vi "Line Configuration Dialog.vi"(8 "error in":errorcluster, 9 "engine configuration in":refnum<class "engine configuration.lvclass">, 10 "tag bus configurable plugin module configuration":refnum<class "OPC UA Client configuration.lvclass">, 11 "Line":T4 {"OPC UA Data Type" items=["Boolean"=1, "SByte"=2, "Byte"=3, "Int16"=4, "UInt16"=5, "Int32"=6, "UInt32"=7, "Int64"=8, "UInt64"=9, "Float"=10, "Double"=11, "String"=12, "DateTime"=13, "ByteString"=15, "Array of Boolean"=101, "Array of SByte"=102, "Array of Byte"=103, "Array of Int16"=104, "Array of UInt16"=105, "Array of Int32"=106, "Array of UInt32"=107, "Array of Int64"=108, "Array of UInt64"=109, "Array of Float"=110, "Array of Double"=111, "Array of String"=112, "Array of DateTime"=113, "Array of ByteString"=115]}) -> (0 "error out":errorcluster, 1 "success":bool, 2 "changed":bool, 3 "Mappings out":T3 {"Line"."OPC UA Data Type" items=["Boolean"=1, "SByte"=2, "Byte"=3, "Int16"=4, "UInt16"=5, "Int32"=6, "UInt32"=7, "Int64"=8, "UInt64"=9, "Float"=10, "Double"=11, "String"=12, "DateTime"=13, "ByteString"=15, "Array of Boolean"=101, "Array of SByte"=102, "Array of Byte"=103, "Array of Int16"=104, "Array of UInt16"=105, "Array of Int32"=106, "Array of UInt32"=107, "Array of Int64"=108, "Array of UInt64"=109, "Array of Float"=110, "Array of Double"=111, "Array of String"=112, "Array of DateTime"=113, "Array of ByteString"=115]})   [LabVIEW 2014, in "OPC UA Client editor node.lvclass"]
uses:
  OPC UA Client editor node.lvclass
  module/configuration/Line.ctl
  <vilib>/NI/Tag Bus Module Framework/channel/TBM channel.lvclass
  module/configuration/OPC UA Data Type.ctl
  Mappings.ctl
  Map.ctl
  permissions.ctl
  <vilib>/NI/Module Execution Interface/Engine Configuration/engine configuration.lvclass
  module/configuration/OPC UA Client configuration.lvclass
  OPC UA DataType Enum.ctl
  <vilib>/NI/Tag Bus Module Framework/channel/TBM channel.lvclass/TBM channel.ctl
  <vilib>/NI/Configuration Framework/serializable configuration/NISE_CEF_serializable configuration.lvclass/NISE_CEF_serializable configuration.ctl
  <vilib>/NI/Tag Bus/tag/tag descriptor.lvclass/tag descriptor.ctl
  <vilib>/NI/Tag Bus/tag/write tag name.vi
  <vilib>/NI/Tag Bus Module Framework/channel/Write channel classification.vi
  <vilib>/NI/Tag Bus/tag/write data type.vi
  <vilib>/NI/Configuration Framework/serializable configuration/Read UID.vi
  <vilib>/NI/Tag Bus Module Framework/channel/Read channel classification.vi
  <vilib>/Utility/LVClass/Get LV Class Name.vi
  <vilib>/NI/Configuration Framework/error generator/NISE_error generator.vi
  <vilib>/NI/Tag Bus/tag/tag descriptor.lvclass
panel:
  in  "OPC Data Type":T1
  in  "Node Path":string="Channel_0"
  out "errors":string
  in  "Access Type":T2
  in  "Tag":i32(listbox)
  in  "Data Type":i32(listbox)
  in  "cancel":bool
  in  "ok":bool
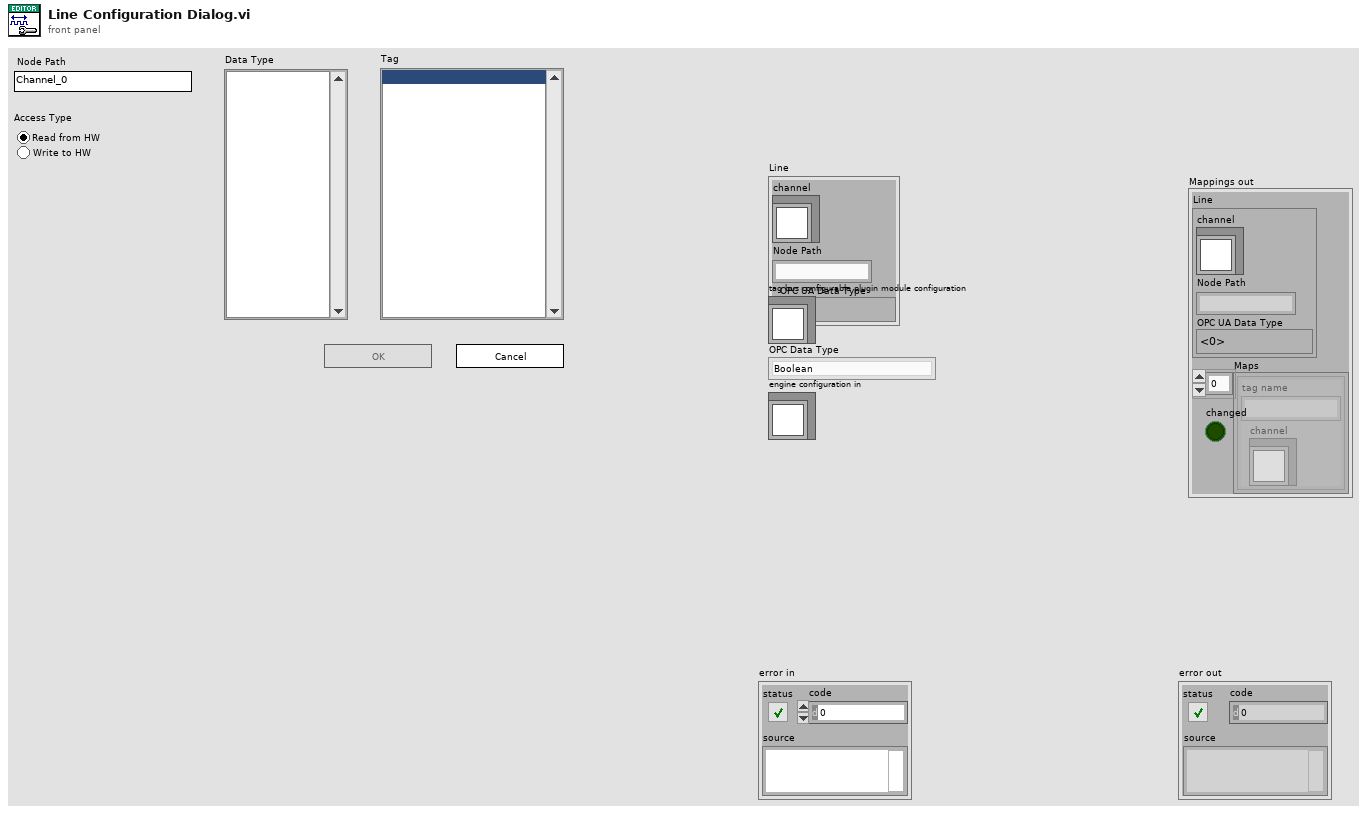
[diagram p1: front panel]
types:
  T1 = typedef "OPC UA Client editor node.lvclass/OPC UA DataType Enum.ctl" = enum16{"Boolean", "SByte", "Byte", "Int16", "UInt16", "Int32", "UInt32", "Int64", "UInt64", "Float", "Double", "String", "DateTime", "ByteString", "Array of Boolean", "Array of SByte", "Array of Byte", "Array of Int16", "Array of UInt16", "Array of Int32", "Array of UInt32", "Array of Int64", "Array of UInt64", "Array of Float", "Array of Double", "Array of String", "Array of DateTime"}
  T2 = typedef "OPC UA Client editor node.lvclass/permissions.ctl" = enum32{"Read from HW", "Write to HW"}
  T3 = typedef "OPC UA Client editor node.lvclass/Mappings.ctl" = cluster{"Line":T4, "Maps":T6[]}
  T4 = typedef "OPC UA Client configuration.lvclass/Line.ctl" = cluster{"channel":refnum<class "TBM channel.lvclass">, "Node Path":string, "OPC UA Data Type":T5}
  T5 = typedef "OPC UA Client configuration.lvclass/OPC UA Data Type.ctl" = u16
  T6 = typedef "OPC UA Client editor node.lvclass/Map.ctl" = cluster{"channel":refnum<class "TBM channel.lvclass">, "tag name":string}
  T7 = typedef "TBM channel.lvclass/channel classification.ctl" = enum16{"input data", "output data", "processing parameter", "processing result"}
  T8 = enum8{"Enabled", "Disabled", "Disabled and Grayed Out"}
  T9 = typedef "tag bus.lvlib/tag descriptor.lvclass/Data Type.ctl" = enum16{"Double", "Single", "I64", "I32", "I16", "I8", "U64", "U32", "U16", "U8", "Boolean", "String", "Array of Double", "Array of Single", "Array of I64", "Array of I32", "Array of I16", "Array of I8", "Array of U64", "Array of U32", "Array of U16", "Array of U8", "Array of Boolean", "Array of String"}
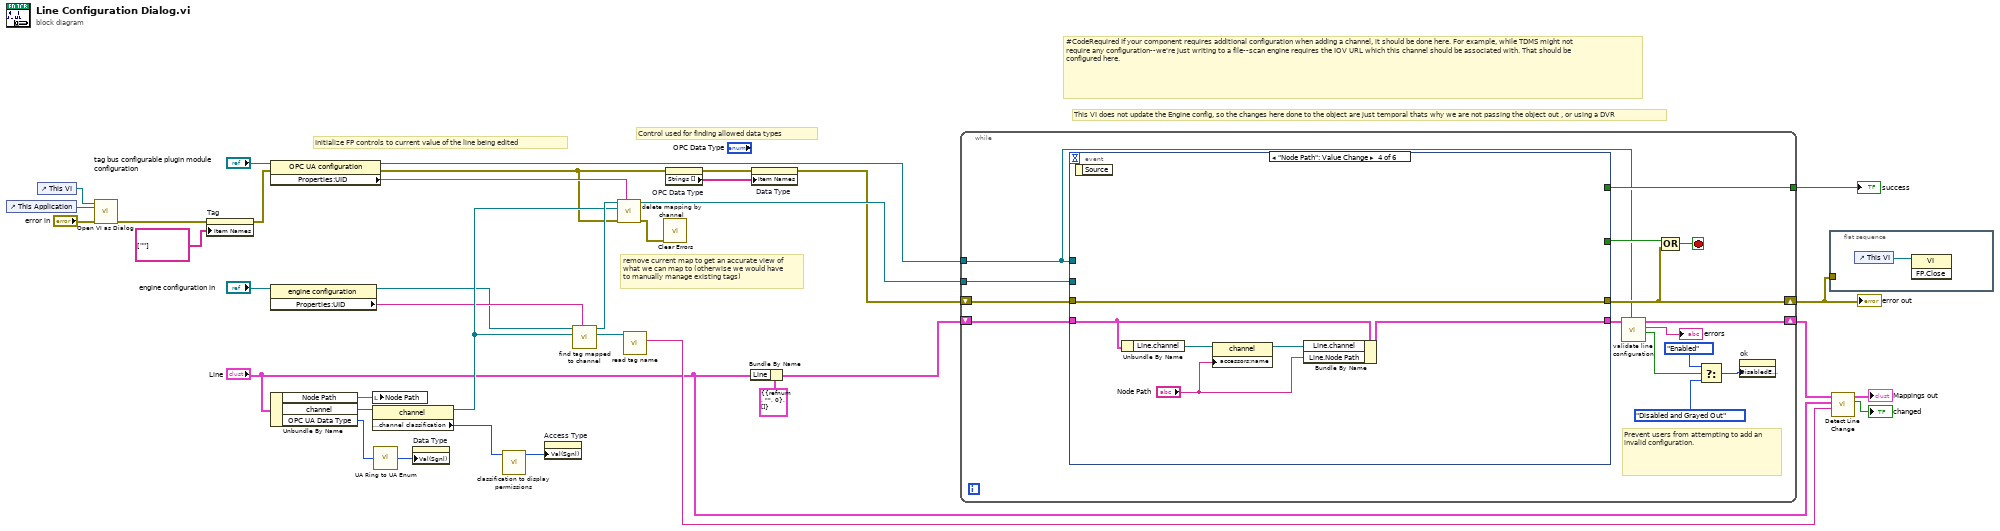
[diagram p0: block diagram]
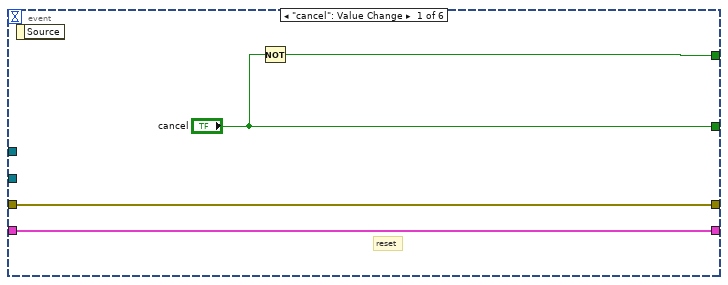
[diagram p2: hidden frame]
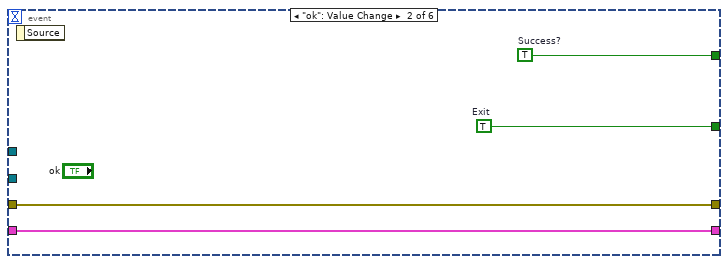
[diagram p3: hidden frame]
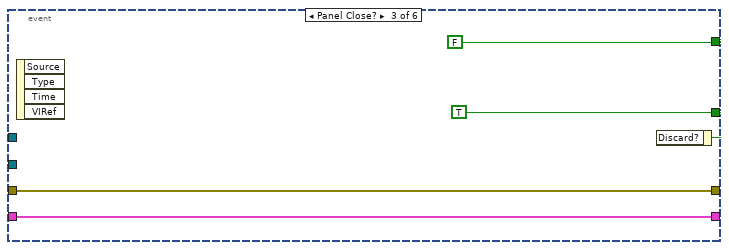
[diagram p4: hidden frame]
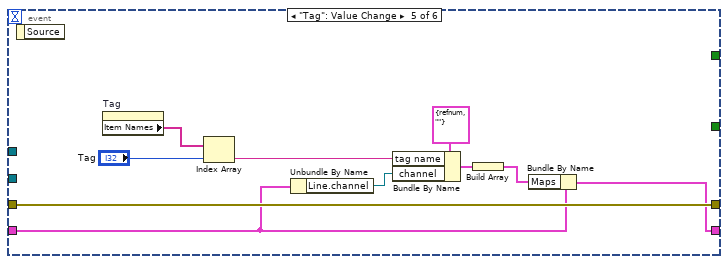
[diagram p5: hidden frame]
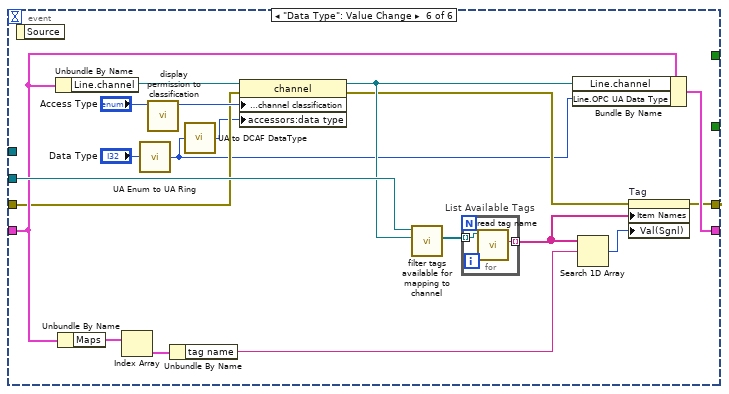
[diagram p6: hidden frame]
diagram:
  # "Control used for finding allowed data types"
  # "Initialize FP controls to current value of the line being edited"
  # "This VI does not update the Engine config, so the changes here done to the object are just temporal thats why we are not passing the object out , or using a DVR"
  # "remove current map to get an accurate view of what we can map to (otherwise we would have to manually manage existing tags)"
  # "#CodeRequired If your component requires additional configuration when adding a channel, it should be done here. For example, while TDMS might not require any configuration--we're just writing to a file--scan engine requires the IOV URL which this channel should be associated with. That should be configured here."
  n1 = control-ref of="This Application"() -> (w33:refnum<vi>)
  n2 = control-ref of="This VI"() -> (w32:refnum<vi>)
  n3 = call "Open VI as Dialog.vi"("error in (no error)"="error in", "This Application"=w33, "VI in"=w32) -> ("error out"=w23:errorcluster)  [unwired: 8 in]
  n4 = property on="Tag" class="LstBox (strict)"(error in=w23, "Item Names"=string[] [""]) -> (error out=w10:errorcluster)  [unwired: 1 in, 1 out]
  n5 = property class="OPC UA configuration"(reference="tag bus configurable plugin module configuration", error in=w10) -> (reference out=w34:refnum<class "OPC UA Client configuration.lvclass">, error out=w6:errorcluster, "Properties:UID"=w8:string)
  n6 = property class="engine configuration"(reference="engine configuration in") -> (reference out=w9:refnum<class "engine configuration.lvclass">, "Properties:UID"=w11:string)  [unwired: 1 in, 1 out]
  n7 = Unbundle By Name("Line") -> ("Node Path"=w21:string, "channel"=w29:refnum<class "TBM channel.lvclass">, "OPC UA Data Type"=w2:T5)
  n8 = local write "Node Path"(w21) -> ()
  n9 = property class="channel"(reference=w29) -> (reference out=w15:refnum<class "TBM channel.lvclass">, "data access:channel classification"=w30:T7)  [unwired: 1 in, 1 out]
  n10 = call "UA Ring to UA Enum.vi"("OPC UA Data Type Ring"=w2) -> ("OPC Data Type Enum"=w3:T1)
  n11 = property on="Data Type" class="LstBox (strict)"("Val(Sgnl)"=w3) -> ()  [unwired: 2 in, 2 out]
  n12 = call "classification to display permissions.vi"("channel classification"=w30) -> ("permissions"=w27:T2)  [unwired: 10 in]
  n13 = property on="Access Type" class="RadioBtnsControl (strict)"("Val(Sgnl)"=w27) -> ()  [unwired: 2 in, 2 out]
  n14 = call <vilib>:"find tag mapped to channel.vi"("owner"=w11, "channel"=w15, "engine configuration in"=w9) -> ("tag"=w14:refnum<class "tag descriptor.lvclass">, "engine configuration out"=w16:refnum<class "engine configuration.lvclass">)  [unwired: 6 in, 1 out]
  n15 = call <vilib>:"delete mapping by channel.vi"("owner ID"=w8, "error in"=w6, "channel"=w15, "engine configuration in"=w16) -> ("error out"=w26:errorcluster, "engine configuration out"=w35:refnum<class "engine configuration.lvclass">)  [unwired: 6 in]
  n16 = call <vilib>:"read tag name.vi"("system tag in"=w14) -> ("name"=w13:string)  [unwired: 8 in, 2 out]
  n17 = call <vilib>:"Clear Errors.vi"("error in (no error)"=w26) -> ()  [unwired: 5 in, 2 out]
  n18 = property on="OPC Data Type" class="Enum (strict)"(error in=w6) -> (error out=w4:errorcluster, "Strings []"=w7:string[])  [unwired: 1 in, 1 out]
  n19 = Bundle By Name(cluster=T3 {"Line"={"channel"=refnum, "Node Path"="", "OPC UA Data Type"=0}, "Maps"=[]} ("Mappings out"), "Line"="Line") -> (w17:T3)
  n20 = property on="Data Type" class="LstBox (strict)"(error in=w4, "Item Names"=w7) -> (error out=w5:errorcluster)  [unwired: 1 in, 1 out]
  n21 = while {
    shift-right: [w43] -> w31
    shift-left: w5 -> [w50]
    tunnel: [w49] -> w36
    shift-right: [w44] -> w20
    shift-left: w17 -> [w46]
    tunnel: w35 -> [w51]
    tunnel: w34 -> [w38]
    stop <- w47 stop-if-true
    # "Prevent users from attempting to add an invalid configuration."
    n22 = event shown="[3] \"Node Path\": Value Change" {
      selector: _ -> [_ _ _ _ _ _]
      dyn-events: _ -> [_ _ _ _ _ _]
      timeout: _ -> [_ _ _ _ _ _]
      tunnel: w51 -> [_ _ _ _ _ w96]
      tunnel: w50 -> [w55 w59 w63 w69 w79 w90]
      tunnel: [w55 w59 w63 w69 w79 w88] -> w43
      tunnel: [w54 w56 FALSE _ _ _] -> w49
      tunnel: ["cancel" w57 w61 _ _ _] -> w48
      tunnel: w46 -> [w52 w58 w60 w67 w73 w94]
      tunnel: [w52 w58 w60 w68 w70 w93] -> w45
      tunnel: w38 -> [_ _ _ _ _ _]
      event "cancel": Value Change {
        # "reset"
        n23 = event-data() -> ()  [unwired: 1 in, 1 out]
        n24 = Not(x="cancel") -> (.not. x?=w54:bool)
      }
      event "ok": Value Change {
        w56 = TRUE  # Success?
        w57 = TRUE  # Exit
        n25 = event-data() -> ()  [unwired: 1 in, 1 out]
      }
      event Panel Close? {
        w61 = TRUE ("cancel")
        n26 = event-data() -> ()  [unwired: 1 in, 4 out]
        n27 = event-data("Discard?"=w61) -> ()  [unwired: 1 in, 1 out]
      }
      event "Node Path": Value Change {
        n28 = event-data() -> ()  [unwired: 1 in, 1 out]
        n29 = Unbundle By Name(w67) -> ("Line.channel"=w66:refnum<class "TBM channel.lvclass">)
        n30 = property class="channel"(reference=w66, "accessors:name"="Node Path") -> (reference out=w65:refnum<class "TBM channel.lvclass">)  [unwired: 1 in, 1 out]
        n31 = Bundle By Name(cluster=w67, "Line.channel"=w65, "Line.Node Path"="Node Path") -> (w68:T3)
      }
      event "Tag": Value Change {
        n32 = event-data() -> ()  [unwired: 1 in, 1 out]
        n33 = property on="Tag" class="LstBox (strict)"() -> ("Item Names"=w77:string[])  [unwired: 2 in, 2 out]
        n34 = Index Array(array=w77, index="Tag") -> (element=w76:string)
        n35 = Unbundle By Name(w73) -> ("Line.channel"=w74:refnum<class "TBM channel.lvclass">)
        n36 = Bundle By Name(cluster=T6 {"channel"=refnum, "tag name"=""} ("Map"), "tag name"=w76, "channel"=w74) -> (w72:T6)
        n37 = Build Array(w72) -> (w71:T6[])
        n38 = Bundle By Name(cluster=w73, "Maps"=w71) -> (w70:T3)
      }
      event "Data Type": Value Change {
        n39 = event-data() -> ()  [unwired: 1 in, 1 out]
        n40 = Unbundle By Name(w94) -> ("Line.channel"=w98:refnum<class "TBM channel.lvclass">)
        n41 = Unbundle By Name(w94) -> ("Maps"=w85:T6[])
        n42 = Index Array(array=w85) -> (element=w84:T6)  [unwired: 1 in]
        n43 = call "UA Enum to UA Ring.vi"("OPC Data Type Enum"="Data Type") -> ("OPC UA Data Type Ring"=w80:T5)
        n44 = call "display permission to classification.vi"("display permissions"="Access Type") -> ("channel classification"=w97:T7)  [unwired: 10 in]
        n45 = Unbundle By Name(w84) -> ("tag name"=w83:string)
        n46 = call "UA to DCAF DataType.vi"("OPC UA Data Type"=w80) -> ("DCAF Datatype"=w81:T9)
        n47 = property class="channel"(reference=w98, error in=w90, "data access:channel classification"=w97, "accessors:data type"=w81) -> (reference out=w95:refnum<class "TBM channel.lvclass">, error out=w89:errorcluster)
        n48 = call-dynamic "filter tags available for mapping to channel.vi"("channel to map to"=w95, "engine configuration in"=w96) -> ("filtered tags"=w92:refnum<class "tag descriptor.lvclass">[])  [unwired: 8 in, 1 out]
        n49 = for "List Available Tags" {
          tunnel: w92 -> [w100] mode=indexing
          tunnel: [w99] -> w87 mode=indexing
          n50 = call <vilib>:"read tag name.vi"("system tag in"=w100) -> ("name"=w99:string)  [unwired: 8 in, 2 out]
        }
        n51 = Bundle By Name(cluster=w94, "Line.channel"=w95, "Line.OPC UA Data Type"=w80) -> (w93:T3)
        n52 = Search 1D Array(1D array=w87, element=w83) -> (index of element=w86:i32)  [unwired: 1 in]
        n53 = property on="Tag" class="LstBox (strict)"(error in=w89, "Item Names"=w87, "Val(Sgnl)"=w86) -> (error out=w88:errorcluster)  [unwired: 1 in, 1 out]
      }
    }
    n54 = call "validate line configuration.vi"("module"=w38, "Mappings in"=w45) -> ("valid?"=w42:bool, "errors"=→"errors":string, "Mappings out"=w44:T3)  [unwired: 7 in]
    n55 = Compound Arithmetic op=OR(w48, w43) -> (w47:bool)
    n56 = Select(t=T8."Enabled" ("Disabled"), s=w42, f=T8."Disabled and Grayed Out") -> (s? t:f=w39:T8)
    n57 = property on="ok" class="Bool"("DisabledEnum"=w39) -> ()  [unwired: 2 in, 2 out]
  }
  "error out" <- w31
  "success" <- w36
  n58 = flat-sequence {
    tunnel: w31 -> [_]
    frame #0 {
      n59 = control-ref of="This VI"() -> (w101:refnum<vi>)
      n60 = invoke class="VI" method="FP.Close"(reference=w101) -> ()  [unwired: 2 in, 3 out]
    }
  }
  n61 = call "Detect Line Change.vi"("Original Tag"=w13, "Original Line"="Line", "Mappings In"=w20) -> ("Changed?"=→"changed":bool, "Mappings Out"=→"Mappings out":T3)  [unwired: 7 in]
